vi "verify parameters in range.vi"(8 "error in (no error)":errorcluster, 11 "Simulated_CCD_Camera in":refnum<class "Simulated Camera.lvclass">) -> (0 "error out":errorcluster, 3 "Simulated_CCD_Camera out":refnum<class "Simulated Camera.lvclass">)   [LabVIEW 2018, in "Simulated Camera.lvclass"]
doc: "Verify if the parameters of the camera are in range\n\nThe operating parameters of the CCDs must be within a predefined range. This function verifies if the values provided for these parameters meet this specification. If not, ACS will not allow to start an exposure."
uses:
  Simulated Camera.lvclass
  Simulated Camera.lvclass/Simulated Camera.ctl
panel:
  out "New CCD Config":T1
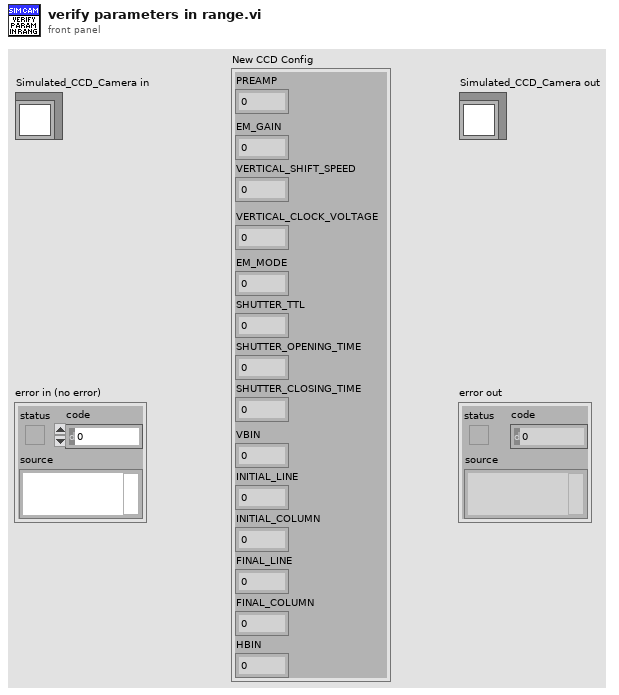
[diagram p1: front panel]
types:
  T1 = cluster{"PREAMP":u16, "EM_GAIN":u16, "VERTICAL_SHIFT_SPEED":u16, "VERTICAL_CLOCK_VOLTAGE":u16, "EM_MODE":u16, "SHUTTER_TTL":u16, "SHUTTER_OPENING_TIME":u16, "SHUTTER_CLOSING_TIME":u16, "VBIN":u16, "INITIAL_LINE":u16, "INITIAL_COLUMN":u16, "FINAL_LINE":u16, "FINAL_COLUMN":u16, "HBIN":u16}
  T2 = cluster{"PREAMP":u16, "READOUT_RATE":u16, "EM_GAIN":u16, "VERTICAL_SHIFT_SPEED":u16, "READ_MODE":u16, "FRAME_TRANSFER":bool, "VERTICAL_CLOCK_VOLTAGE":u16, "ACQUISITION_MODE":u16, "AD_CHANNEL":u16, "EM_MODE":u16, "SHUTTER_TTL":u16, "SHUTTER_OPENING_TIME":u16, "SHUTTER_CLOSING_TIME":u16, "SHUTTER_MODE":u16, "TRIGGER_MODE":u16, "VBIN":u16, "INITIAL_LINE":u16, "INITIAL_COLUMN":u16, "FINAL_LINE":u16, "FINAL_COLUMN":u16, "HBIN":u16}
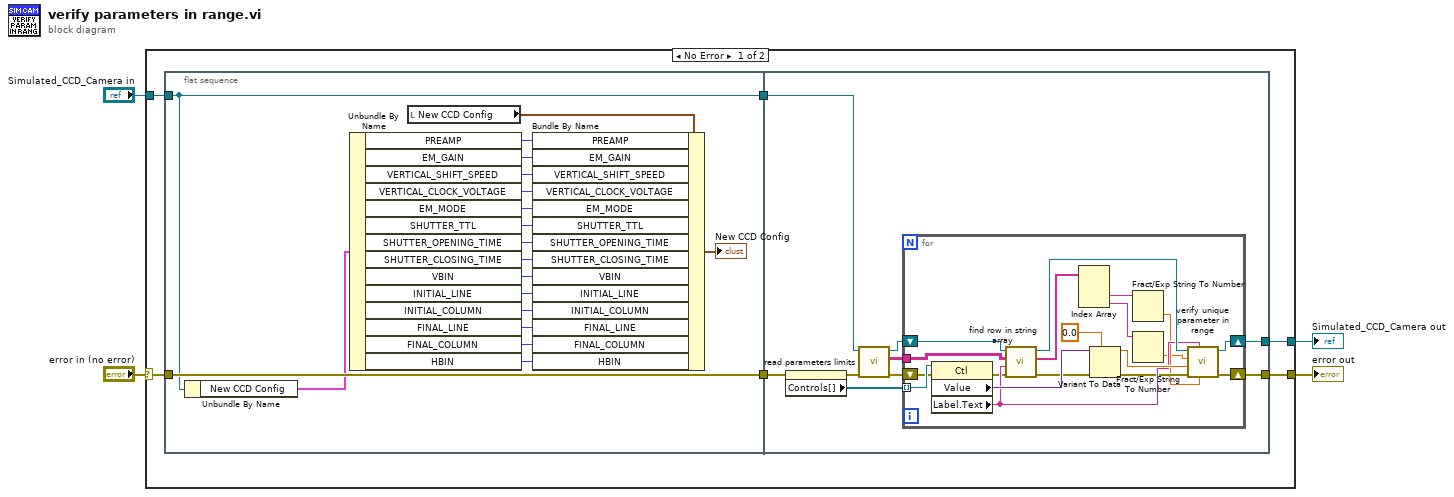
[diagram p0: block diagram]
diagram:
  n1 = case shown="No Error" "error in (no error)" {
    selector: "error in (no error)" -> [w8 w59]
    tunnel: [w10 w59] -> w3
    tunnel: [w9 w58] -> w2
    tunnel: "Simulated_CCD_Camera in" -> [w7 w58]
    frame No Error {
      n2 = flat-sequence {
        tunnel: w7 -> [w28]
        tunnel: w8 -> [w29]
        tunnel: [w29] -> w6
        tunnel: [w28] -> w5
        tunnel: [w38] -> w10
        tunnel: [w36] -> w9
        tunnel: w6 -> [w31]
        tunnel: w5 -> [w32]
        frame #0 {
          n3 = Unbundle By Name(w28) -> ("New CCD Config"=w13:T2)
          n4 = Unbundle By Name(w13) -> ("PREAMP"=w14:u16, "EM_GAIN"=w15:u16, "VERTICAL_SHIFT_SPEED"=w16:u16, "VERTICAL_CLOCK_VOLTAGE"=w17:u16, "EM_MODE"=w18:u16, "SHUTTER_TTL"=w19:u16, "SHUTTER_OPENING_TIME"=w20:u16, "SHUTTER_CLOSING_TIME"=w21:u16, "VBIN"=w22:u16, "INITIAL_LINE"=w23:u16, "INITIAL_COLUMN"=w24:u16, "FINAL_LINE"=w25:u16, "FINAL_COLUMN"=w26:u16, "HBIN"=w27:u16)
          n5 = local read "New CCD Config"() -> (w11:T1)
          n6 = Bundle By Name(cluster=w11, "PREAMP"=w14, "EM_GAIN"=w15, "VERTICAL_SHIFT_SPEED"=w16, "VERTICAL_CLOCK_VOLTAGE"=w17, "EM_MODE"=w18, "SHUTTER_TTL"=w19, "SHUTTER_OPENING_TIME"=w20, "SHUTTER_CLOSING_TIME"=w21, "VBIN"=w22, "INITIAL_LINE"=w23, "INITIAL_COLUMN"=w24, "FINAL_LINE"=w25, "FINAL_COLUMN"=w26, "HBIN"=w27) -> (→"New CCD Config":T1)
        }
        frame #1 {
          n7 = property on="New CCD Config" class="Clust (strict)"(error in=w31) -> (error out=w30:errorcluster, "Controls[]"=w37:refnum<vi>[])  [unwired: 1 in, 1 out]
          n8 = call "read parameters limits.vi"("error in (no error)"=w30, "Simulated_CCD_Camera in"=w32) -> ("error out"=w35:errorcluster, "limit values spreadsheet"=w34:string[][], "Simulated_CCD_Camera out"=w33:refnum<class "Simulated Camera.lvclass">)  [unwired: 7 in]
          n9 = for {
            shift-right: [w57] -> w38
            shift-left: w35 -> [w41]
            tunnel: w37 -> [w56] mode=indexing
            tunnel: w34 -> [w51]
            shift-right: [w52] -> w36
            shift-left: w33 -> [w49]
            n10 = property class="Ctl"(reference=w56, error in=w41) -> (error out=w43:errorcluster, "Value"=w55:variant, "Label.Text"=w45:string)  [unwired: 1 out]
            n11 = call "find row in string array.vi"("error in (no error)"=w43, "parameter name"=w45, "limit values"=w51, "Simulated_CCD_Camera in"=w49) -> ("error out"=w42:errorcluster, "row"=w50:string[], "Simulated_CCD_Camera out"=w48:refnum<class "Simulated Camera.lvclass">)  [unwired: 5 in]
            n12 = Index Array(array=w50) -> (element #2=w47:string, element #3=w46:string)  [unwired: 3 in, 1 out]
            n13 = Variant To Data(error in=w42, type=0.0, Variant=w55) -> (data=w53:dbl, error out=w44:errorcluster)
            n14 = Fract/Exp String To Number(string=w47) -> (number=w40:dbl)  [unwired: 3 in, 1 out]
            n15 = Fract/Exp String To Number(string=w46) -> (number=w39:dbl)  [unwired: 3 in, 1 out]
            n16 = call "verify unique parameter in range.vi"("lower limit"=w40, "parameter name"=w45, "error in (no error)"=w44, "value"=w53, "upper limit"=w39, "Simulated_CCD_Camera in"=w48) -> ("error out"=w57:errorcluster, "Simulated_CCD_Camera out"=w52:refnum<class "Simulated Camera.lvclass">)  [unwired: 4 in]
          }
        }
      }
    }
    frame Error {
    }
  }
  "error out" <- w3
  "Simulated_CCD_Camera out" <- w2
